vi "XML Create Spec Tag.vi"() -> (3 "XML Spec tag":string)   [LabVIEW 2012]
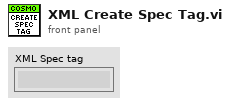
[diagram p1: front panel]
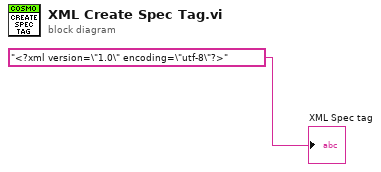
[diagram p0: block diagram]
diagram:
  "XML Spec tag" <- "<?xml version=\"1.0\" encoding=\"utf-8\"?>"
